vi "RPC Method Query.vi"(8 "error in (no error)":errorcluster, 11 "OOP Server in":refnum<class "OOP Query Server.lvclass">) -> (0 "error out":errorcluster)   [LabVIEW 2019, in "OOP Query Server.lvlib" / "OOP Query Server.lvclass"]
uses:
  OOP Query Server.lvclass
  RPC Messages/QueryResponse/QueryResponse_Data.ctl
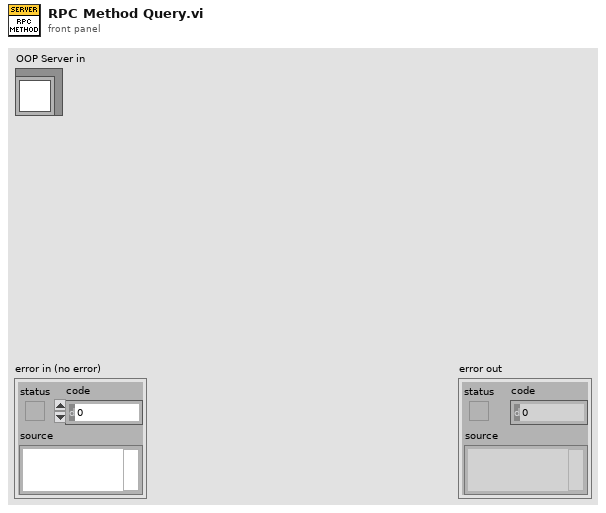
[diagram p1: front panel]
types:
  T1 = typedef "OOP Query Server.lvlib/OOP Query Server.lvclass/QueryResponse_Data.ctl" = cluster{"message":string, "status":i32}
  T2 = typedef "OOP Query Server.lvlib/OOP Query Server.lvclass/Server Internal UEs.ctl" = cluster{"Invoke Internal UE":refnum<user-event>, "Query Internal UE":refnum<user-event>, "Register Internal UE":refnum<user-event>}
  T3 = typedef "OOP Query Server.lvlib/OOP Query Server.lvclass/Server gRPC UEs.ctl" = cluster{"Invoke gRPC UE":refnum<user-event>, "Query gRPC UE":refnum<user-event>, "Register gRPC UE":refnum<user-event>}
  T4 = typedef "OOP Query Server.lvlib/gprc-lvsupport.lvlib/grpcId.ctl" = u64
  T5 = typedef "OOP Query Server.lvlib/OOP Query Server.lvclass/QueryRequest_Data.ctl" = cluster{"query":string}
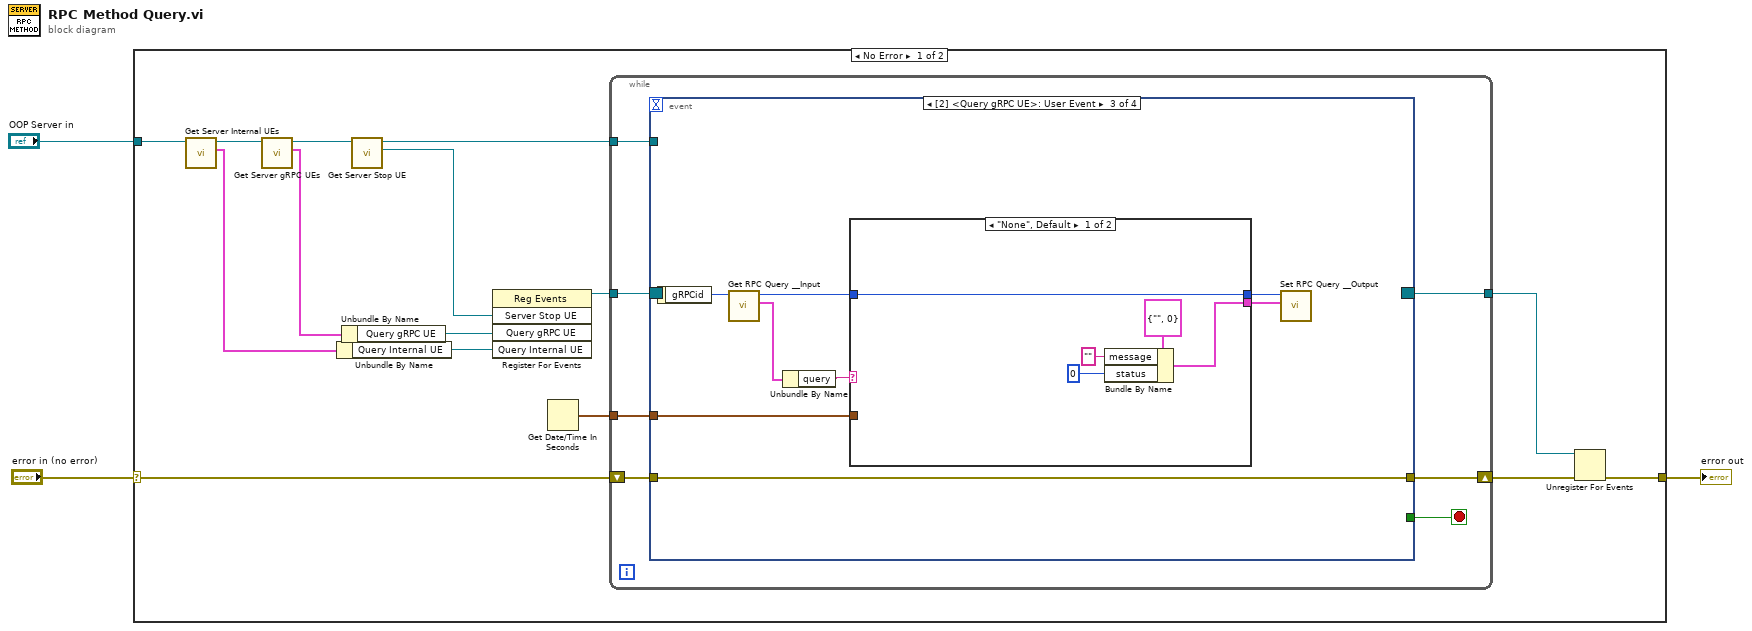
[diagram p0: block diagram]
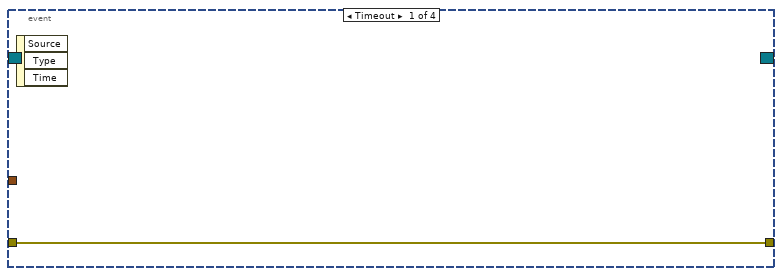
[diagram p2: hidden frame]
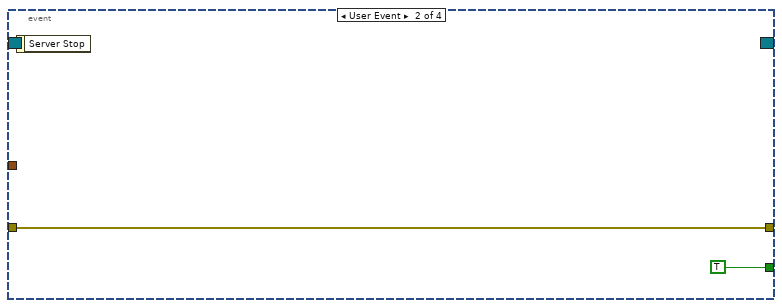
[diagram p3: hidden frame]
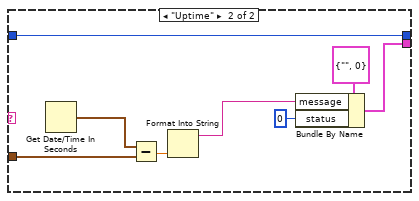
[diagram p4: hidden frame]
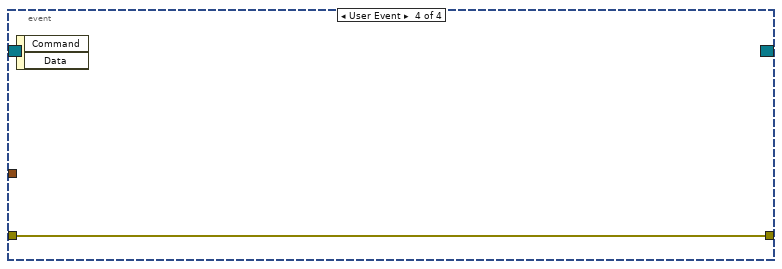
[diagram p5: hidden frame]
diagram:
  n1 = case shown="No Error" "error in (no error)" {
    selector: "error in (no error)" -> [w13 w51]
    tunnel: [w11 w51] -> w2
    tunnel: "OOP Server in" -> [w15 _]
    frame No Error {
      n2 = call "Get Server Internal UEs.vi"("OOP Server in"=w15) -> ("Server Internal UEs"=w7:T2, "OOP Server out"=w14:refnum<class "OOP Query Server.lvclass">)  [unwired: 9 in]
      n3 = call "Get Server gRPC UEs.vi"("OOP Server in"=w14) -> ("Server gRPC UEs"=w9:T3, "OOP Server out"=w18:refnum<class "OOP Query Server.lvclass">)  [unwired: 9 in]
      n4 = Unbundle By Name ("Unbundle Internal UE")(w7) -> ("Query Internal UE"=w6:refnum<user-event>)
      n5 = Unbundle By Name ("Unbundle gRPC UE")(w9) -> ("Query gRPC UE"=w8:refnum<user-event>)
      n6 = call "Get Server Stop UE.vi"("OOP Server in"=w18) -> ("Server Stop UE"=w17:refnum<user-event>, "OOP Server out"=w5:refnum<class "OOP Query Server.lvclass">)  [unwired: 9 in]
      n7 = register-events(w17, w8, w6) -> (reference out=w16:refnum<event-registration>)  [unwired: 2 in, 1 out]
      n8 = Get Date/Time In Seconds() -> (seconds since 1Jan1904=w4:timestamp)
      n9 = while {
        tunnel: w16 -> [w25]
        tunnel: [w21] -> w10
        shift-right: [w22] -> w12
        shift-left: w13 -> [w23]
        tunnel: w5 -> [w20]
        tunnel: w4 -> [w19]
        stop <- w24 stop-if-true
        n10 = event "RPC Method Event Structure" shown="[2] <Query gRPC UE>: User Event" {
          selector: w25 -> [_ _ _ _]
          dyn-events: [_ _ _ _] -> w21
          timeout: _ -> [_ _ _ _]
          tunnel: [_ TRUE _ _] -> w24
          tunnel: w23 -> [w26 w27 w29 w50]
          tunnel: [w26 w27 w29 w50] -> w22
          tunnel: w20 -> [_ _ _ _]
          tunnel: w19 -> [_ _ w31 _]
          event Timeout {
            n11 = event-data() -> ()  [unwired: 1 in, 3 out]
          }
          event User Event {
            n12 = event-data() -> ()  [unwired: 1 in, 1 out]
          }
          event User Event {
            n13 = event-data() -> ("gRPCid"=w36:T4)  [unwired: 1 in]
            n14 = call "Get RPC Query __Input.vi"("gRPCid in"=w36) -> ("Message Data"=w35:T5, "gRPCid out"=w33:T4)  [unwired: 8 in, 1 out]
            n15 = Unbundle By Name(w35) -> ("query"=w34:string)
            n16 = case shown="\"None\", Default" w34 {
              tunnel: w33 -> [w41 w49]
              tunnel: [w41 w49] -> w32
              tunnel: w31 -> [_ w45]
              tunnel: [w38 w42] -> w30
              frame "None", Default {
                n17 = Bundle By Name(cluster=T1 {"message"="", "status"=0} ("Message Data"), "message"="", "status"=0) -> (w38:T1)
              }
              frame "Uptime" {
                n18 = Get Date/Time In Seconds() -> (seconds since 1Jan1904=w47:timestamp)
                n19 = Subtract(x=w47, y=w45) -> (x-y=w46:dbl)
                n20 = Format Into String(w46) -> (resulting string=w44:string)  [unwired: 3 in, 1 out]
                n21 = Bundle By Name(cluster=T1 {"message"="", "status"=0} ("Message Data"), "message"=w44, "status"=0) -> (w42:T1)
              }
            }
            n22 = call "Set RPC Query __Output.vi"("Message Data"=w30, "gRPCid in"=w32) -> ()  [unwired: 9 in, 1 out]
          }
          event User Event {
            n23 = event-data() -> ()  [unwired: 1 in, 2 out]
          }
        }
      }
      n24 = Unregister For Events(event registration refnum=w10, error in=w12) -> (error out=w11:errorcluster)
    }
    frame Error {
    }
  }
  "error out" <- w2
